vi "Stop Core.vi"(10 "final error code":i32, 11 "Log in":refnum<class "Log.lvclass">) -> (3 "Log out":refnum<class "Log.lvclass">)   [LabVIEW 2015, in "AMS UI.lvlib" / "Log.lvclass"]
doc: "(<B>Filename</B>: Actor Framework.lvlib:Actor.lvclass:Stop Core.vi)\n\nDefines what the actor does before it stops. Use the <B>final error code</B> input to determine whether the actor shut down in response to an error.\n\nBy default, this method does nothing. A descendant class may override it to define behavior, such as shutting down any processes the actor initiated in its override of the Actor Core method."
uses:
  Log.lvclass
  Log.lvclass/Log.ctl
  AMS Gas Actor/AMS Gas Actor.lvclass
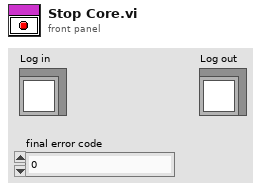
[diagram p1: front panel]
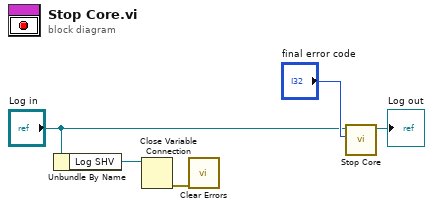
[diagram p0: block diagram]
diagram:
  n1 = Unbundle By Name("Log in") -> ("Log SHV"=w2:refnum<k21>)
  n2 = Close Variable Connection(11:w2) -> (0:w1:errorcluster)  [unwired: 1 in]
  n3 = call <vilib>:"Clear Errors.vi"("error in (no error)"=w1) -> ()  [unwired: 5 in, 2 out]
  n4 = call-parent "Stop Core.vi"("final error code"="final error code", "AMS Gas Actor in"="Log in") -> ("AMS Gas Actor out"=→"Log out":refnum<class "Log.lvclass">)  [unwired: 9 in]
